vi "Pull_Up_Down_Zero.vi"(6 "Keithley 2400 Actuator Pull-DN PS":refnum<visa-resource-name>="GPIB0::10::INSTR", 8 "error in (no error)":errorcluster, 9 "Current Limit Pull-DN (A)":dbl=0.1, 10 "Current Limit Pull-Up(A)":dbl=0.1, 11 "Keithley 2400 Actuator Pull-Up PS":refnum<visa-resource-name>="GPIB0::2::INSTR") -> (0 "error out":errorcluster)   [LabVIEW 2017]
uses:
  Instrument Drivers/keithley_24xx/Keithley 24XX/Keithley 24XX.lvlib
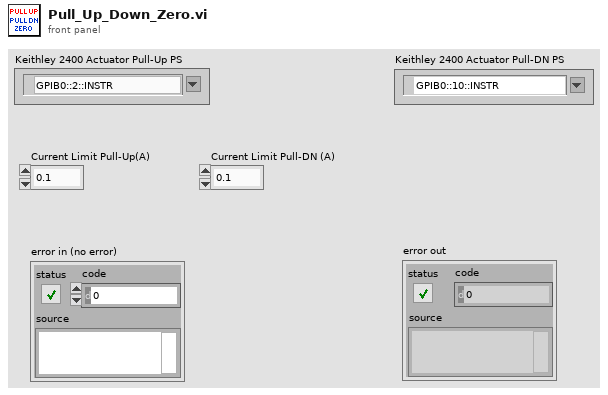
[diagram p1: front panel]
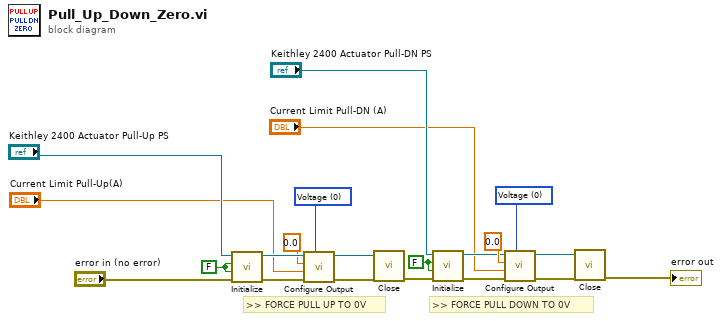
[diagram p0: block diagram]
diagram:
  w8 = FALSE ("ID Query (True)")
  w9 = u16 0 items=["Voltage", "Current"] ("Source Mode  (0: Voltage)")
  w20 = u16 0 items=["Voltage", "Current"] ("Source Mode  (0: Voltage)")
  w21 = FALSE ("Reset (True)")
  # ">> FORCE PULL DOWN TO 0V"
  # ">> FORCE PULL UP TO 0V"
  n1 = call "Initialize.vi"("error in (no error)"="error in (no error)", "Reset (True)"=w21, "ID Query (True)"=w21, "VISA resource name"="Keithley 2400 Actuator Pull-Up PS") -> ("error out"=w19:errorcluster, "VISA resource name out"=w18:refnum<visa-resource-name>)  [unwired: 6 in]
  n2 = call "Configure Output.vi"("Source Mode  (0: Voltage)"=w20, "error in (no error)"=w19, "Compliance  Level (0.1)"="Current Limit Pull-Up(A)", "Output Level (0)"=0.0, "VISA resource name"=w18) -> ("error out"=w15:errorcluster, "VISA resource name out"=w16:refnum<visa-resource-name>)  [unwired: 5 in]
  n3 = call "Close.vi"("error in (no error)"=w15, "VISA resource name"=w16) -> ("error out"=w7:errorcluster)  [unwired: 9 in]
  n4 = call "Initialize.vi"("error in (no error)"=w7, "Reset (True)"=w8, "ID Query (True)"=w8, "VISA resource name"="Keithley 2400 Actuator Pull-DN PS") -> ("error out"=w10:errorcluster, "VISA resource name out"=w11:refnum<visa-resource-name>)  [unwired: 6 in]
  n5 = call "Configure Output.vi"("Source Mode  (0: Voltage)"=w9, "error in (no error)"=w10, "Compliance  Level (0.1)"="Current Limit Pull-DN (A)", "Output Level (0)"=0.0, "VISA resource name"=w11) -> ("error out"=w14:errorcluster, "VISA resource name out"=w13:refnum<visa-resource-name>)  [unwired: 5 in]
  n6 = call "Close.vi"("error in (no error)"=w14, "VISA resource name"=w13) -> ("error out"=→"error out":errorcluster)  [unwired: 9 in]
